vi "set_z_voltage.vi"(8 "error in (no error)":errorcluster, 10 "Z voltage (bits)":i16, 11 "PI P123.01 & PiezoDrive TD250 & NI USB 7855R in":refnum<class "PI P123.01 & PiezoDrive TD250 & NI USB 7855R.lvclass">) -> (0 "error out":errorcluster, 3 "PI P123.01 & PiezoDrive TD250 & NI USB 7855R out":refnum<class "PI P123.01 & PiezoDrive TD250 & NI USB 7855R.lvclass">)   [LabVIEW 2020, in "PI P123.01 & PiezoDrive TD250 & NI USB 7855R.lvclass"]
uses:
  PI P123.01 & PiezoDrive TD250 & NI USB 7855R.lvclass
  <vilib>/FPGAPlugInAG/USB-7855R/niLvFpga_Open_USB-7855R.vi
  <vilib>/rvi/interface/common/dynamic/niFpgaDynamicAddResources.vi
  <vilib>/Utility/error.llb/Error Cluster From Error Code.vi
  <vilib>/rvi/errors/niLvFpgaAdjustHostInterfaceError.vi
  PZT/PZT.lvclass
  <vilib>/rvi/interface/nirviOpenFPGA/nirviOpenFPGA.xnode
  FPGA Bitfiles/afmcontrol_FPGATarget_FPGAmain_od6Q9YeVPLc.lvbitx
  FPGA main.vi
  <vilib>/rvi/interface/nirviReadWriteControl/nirviReadWriteControl.xnode
  <vilib>/rvi/interface/Simulation/niFpgaSimulationCallBeginRW.vi
  NiFpgaLv.dll
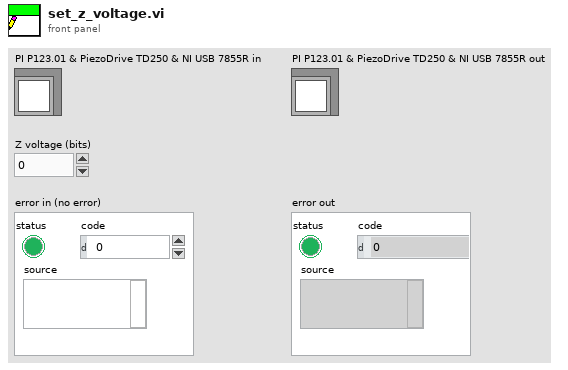
[diagram p1: front panel]
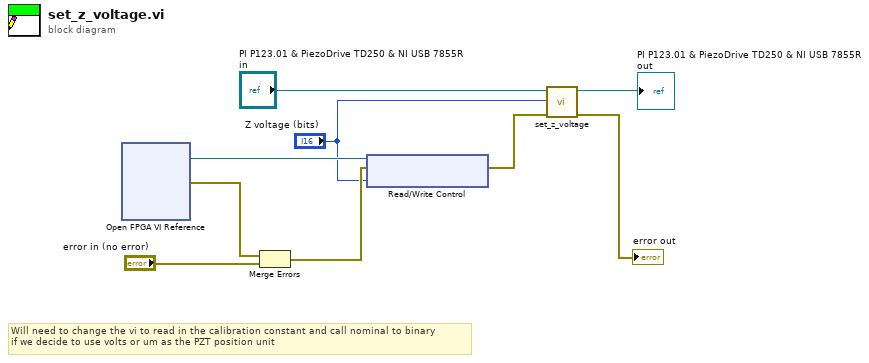
[diagram p0: block diagram]
diagram:
  # "Will need to change the vi to read in the calibration constant and call nominal to binary\nif we decide to use volts or um as the PZT position unit"
  n1 = xnode "Open FPGA VI Reference"() -> ("FPGA VI Reference Out"=w8:refnum<k20>, "error out"=w9:errorcluster)  [unwired: 2 in]
  n2 = Merge Errors(w9, "error in (no error)") -> (w7:errorcluster)
  n3 = xnode "Read/Write Control"("FPGA VI Reference In"=w8, "error in"=w7, "PZT Z Control (Bits)"="Z voltage (bits)") -> ("error out"=w5:errorcluster)  [unwired: 1 out]
  n4 = call-parent "set_z_voltage.vi"("error in (no error)"=w5, "Z voltage (bits)"="Z voltage (bits)", "PZT in"="PI P123.01 & PiezoDrive TD250 & NI USB 7855R in") -> ("error out"=→"error out":errorcluster, "PZT out"=→"PI P123.01 & PiezoDrive TD250 & NI USB 7855R out":refnum<class "PI P123.01 & PiezoDrive TD250 & NI USB 7855R.lvclass">)  [unwired: 7 in]
